vi "Add AO Register.vi"(8 "error in (no error)":errorcluster, 9 "Mapping":T1={"DataType"=enum."U16", "Unit ID"=0, "Starting Address"=0, "Sub-Index (Bool)"=0, "VS Reference"=0} {"VS Reference" format="%.0x"}, 10 "Label":string="Holding Register", 11 "Node Ref In":T3 format="%.0x") -> (0 "error out":errorcluster, 2 "Channel Ref out":T3 format="%.0x", 3 "Node Ref out":T3 format="%.0x")   [LabVIEW 2021, in "Modbus Master System Explorer.lvlib"]
uses:
  Modbus Master System Explorer.lvlib
  <vilib>/NI VeriStand/Custom Device API/Custom Device Item Ref.ctl
  Shared/Controls/Data Model/Mapping.ctl
  Shared/Controls/Data Model/DataType.ctl
  <vilib>/NI VeriStand/Custom Device API/Custom Device Channel.ctl
  <vilib>/NI VeriStand/Custom Device API/Custom Device Channel Type.ctl
  Modbus Type.ctl
  Radix.ctl
  Shared/Constants.vi
  <vilib>/NI VeriStand/Custom Device API/Custom Device API.lvlib
  Shared/Modbus Master Shared.lvlib
  <vilib>/NI VeriStand/Custom Device Tools/Custom Device Utility Library/Custom Device Utility Library.lvlib
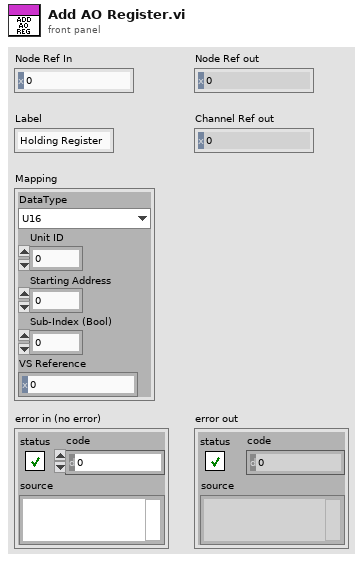
[diagram p1: front panel]
types:
  T1 = typedef "Modbus Master Shared.lvlib/Mapping.ctl" = cluster{"DataType":T2, "Unit ID":u8, "Starting Address":u16, "Sub-Index (Bool)":u16, "VS Reference":T3}
  T2 = typedef "Modbus Master Shared.lvlib/DataType.ctl" = enum16{"Double", "Single", "I64", "I32", "I16", "I8", "U64", "U32", "U16", "U8", "Boolean"}
  T3 = typedef "Custom Device API.lvlib/Custom Device Item Ref.ctl" = u64
  T4 = typedef "Modbus Master System Explorer.lvlib/Radix.ctl" = enum32{"Decimal", "Hexidecimal"}
  T5 = typedef "Custom Device API.lvlib/Custom Device Channel Type.ctl" = enum16{"Input", "Output"}
  T6 = typedef "Modbus Master Shared.lvlib/Modbus Type.ctl" = enum16{"Coil", "Discrete Input", "Holding Register", "Input Register"}
  T7 = typedef "Custom Device API.lvlib/Custom Device Channel.ctl" = cluster{"Type":T5, "Units":string, "Default Value":dbl, "Faultable":bool, "Scalable":bool}
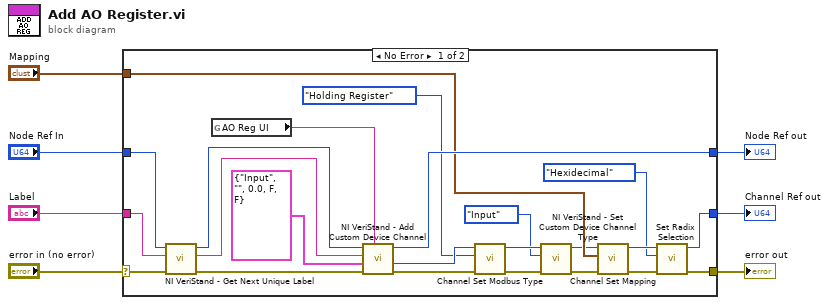
[diagram p0: block diagram]
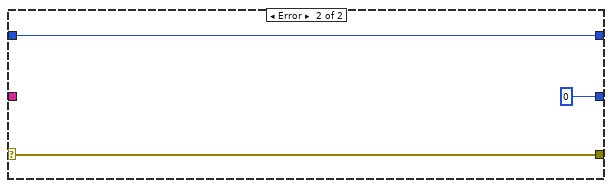
[diagram p2: hidden frame]
diagram:
  n1 = case shown="No Error" "error in (no error)" {
    selector: "error in (no error)" -> [w24 w32]
    tunnel: "Node Ref In" -> [w26 w33]
    tunnel: [w23 w33] -> w5
    tunnel: [w9 w32] -> w4
    tunnel: [w10 T3 0 ("Item Ref out")] -> w3
    tunnel: "Label" -> [w22 _]
    tunnel: "Mapping" -> [w21 _]
    frame No Error {
      n2 = call <vilib>:"NI VeriStand - Get Next Unique Label.vi"("error in (no error)"=w24, "Label"=w22, "Parent Ref in"=w26) -> ("error out"=w28:errorcluster, "Label out"=w29:string, "Parent Ref dup"=w27:T3)  [unwired: 5 in, 1 out]
      n3 = global read "Constants.vi" "AO Reg UI"() -> (w25:string)
      n4 = call <vilib>:"NI VeriStand - Add Custom Device Channel.vi"("GUID (Default Channel)"=w25, "error in (no error)"=w28, "Channel"=T7 {"Type"=enum."Input", "Units"="", "Default Value"=0.0, "Faultable"=FALSE, "Scalable"=FALSE}, "Channel Name"=w29, "Parent Ref in"=w27) -> ("error out"=w19:errorcluster, "Channel Ref"=w20:T3, "Parent Ref out"=w23:T3)  [unwired: 3 in, 1 out]
      n5 = call "Channel Set Modbus Type.vi"("error in (no error)"=w19, "Type"=Modbus_Type."Holding Register", "Channel Ref"=w20) -> ("error out"=w15:errorcluster, "Item Ref out"=w17:T3)  [unwired: 7 in]
      n6 = call <vilib>:"NI VeriStand - Set Custom Device Channel Type.vi"("error in (no error)"=w15, "Type"=Custom_Device_Channel_Type."Input", "Channel Ref in"=w17) -> ("error out"=w14:errorcluster, "Channel Ref out"=w16:T3)  [unwired: 7 in]
      n7 = call "Channel Set Mapping.vi"("error in (no error)"=w14, "Mapping"=w21, "Item Ref in"=w16) -> ("error out"=w11:errorcluster, "Item Ref out"=w12:T3)  [unwired: 7 in]
      n8 = call "Set Radix Selection.vi"("error in (no error)"=w11, "Radix"=Radix."Hexidecimal", "Item Ref in"=w12) -> ("error out"=w9:errorcluster, "Item Ref out"=w10:T3)  [unwired: 7 in]
    }
    frame Error {
    }
  }
  "error out" <- w4
  "Node Ref out" <- w5
  "Channel Ref out" <- w3
